vi "CRYUpdate Graph Window.vi"(8 "sOption":string="Update", 9 "Index":i32[](array[numeric]), 10 "Del/Update Names":string[](array[string]), 11 "Type":enum16{"Curves", "Values", "Results", "WFM"}(ring)) -> ()   [LabVIEW 2013]
uses:
  CRYCurveLibrary/Global/CRYCurve Library Global.vi
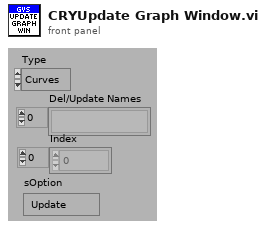
[diagram p1: front panel]
types:
  T1 = cluster{"Curve Index":i32[], "Value Index":i32[], "Result Index":i32[], "WFM Index":i32[], "Curve Names":string[], "Value Names":string[], "Result Names":string[], "WFM Names":string[]}
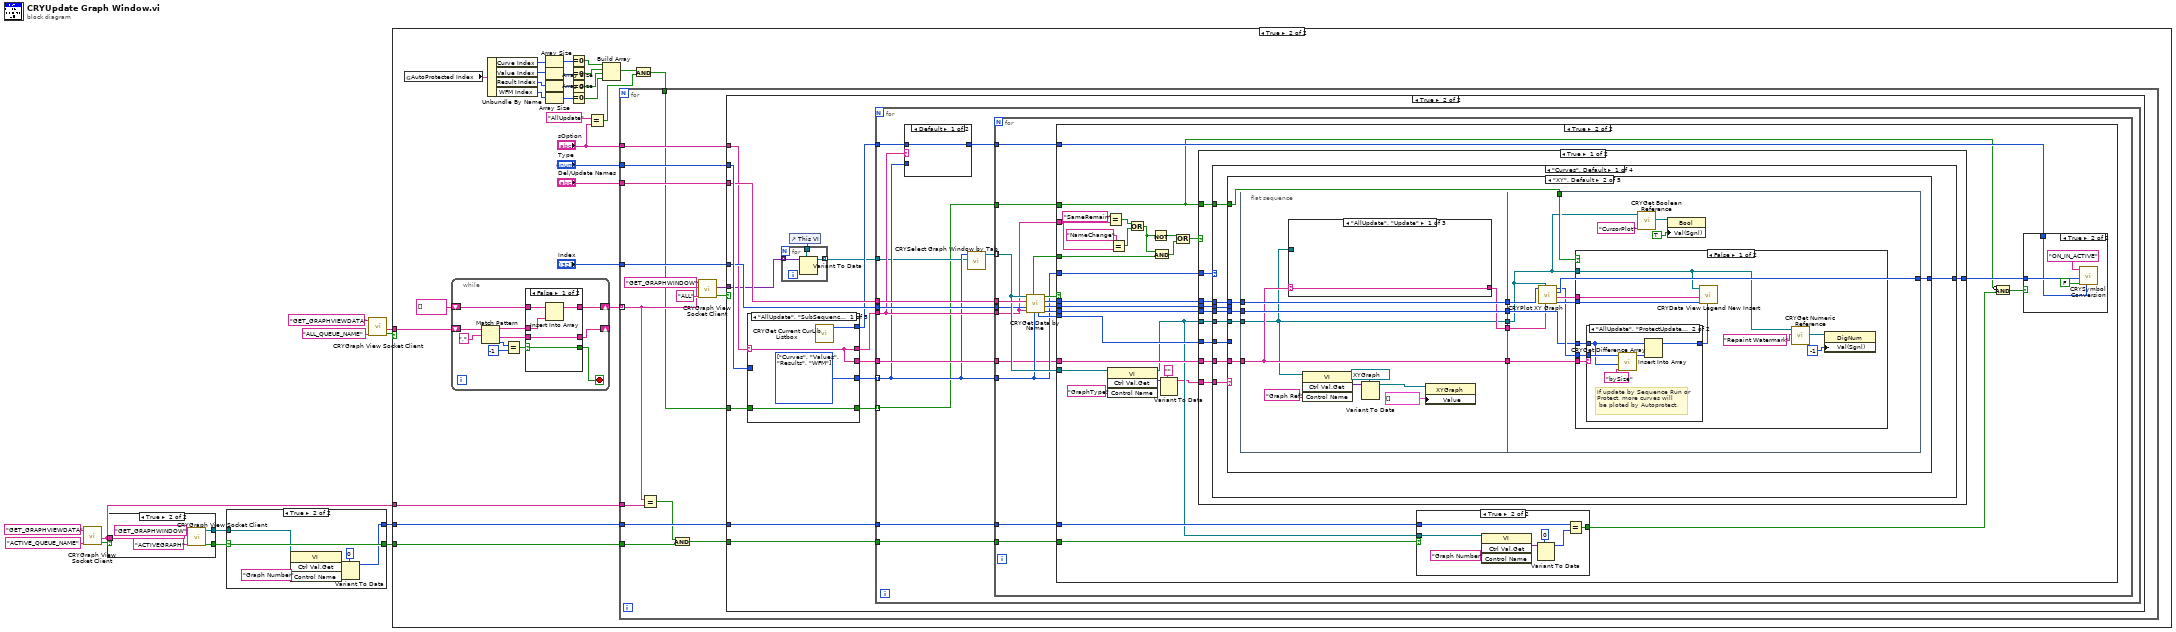
[diagram p0: block diagram]
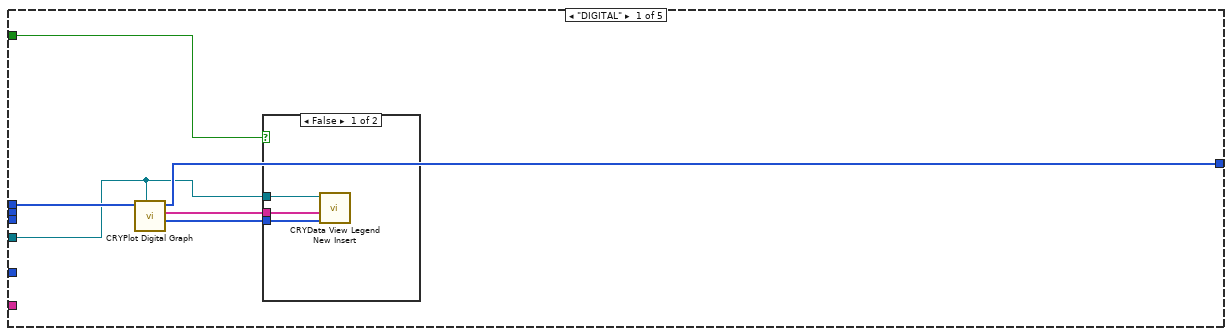
[diagram p10: hidden frame]
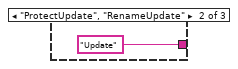
[diagram p12: hidden frame]
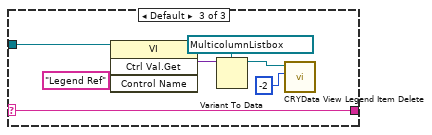
[diagram p13: hidden frame]
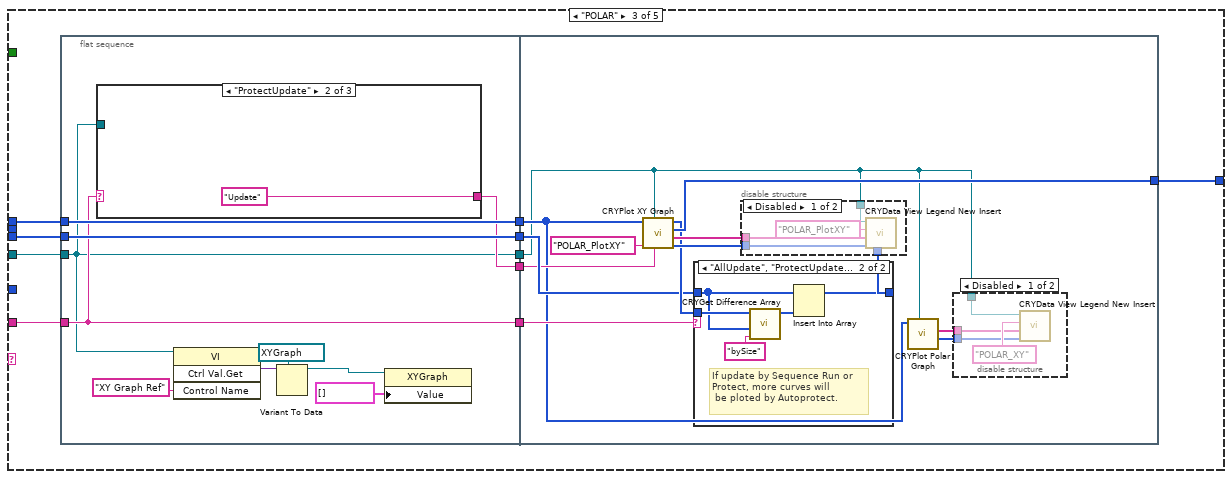
[diagram p16: hidden frame]
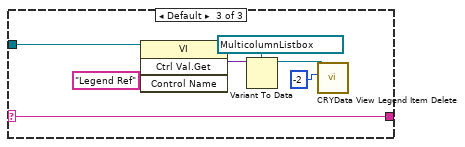
[diagram p18: hidden frame]
diagram:
  n1 = call "CRYGraph View Socket Client.vi"("sOption"="ACTIVE_QUEUE_NAME", "sAction"="GET_GRAPHVIEWDATA") -> ("bResult Out"=w6:bool, "sData Out"=w1:string)  [unwired: 6 in, 2 out]
  n2 = case shown="True" w6 {
    selector: w6 -> [w13 _]
    tunnel: w1 -> [_ w16]
    tunnel: [w13 w15] -> w5
    tunnel: [_ w14] -> w4
    frame False {
    }
    frame True {
      n3 = call "CRYGraph View Socket Client.vi"("sOption"="ACTIVEGRAPH", "sData"=w16, "sAction"="GET_GRAPHWINDOW") -> ("bResult Out"=w15:bool, "pVI Out"=w14:refnum<vi>)  [unwired: 5 in, 2 out]
    }
  }
  n4 = case shown="True" w5 {
    selector: w5 -> [w19 w25]
    tunnel: w4 -> [_ w21]
    tunnel: [_ w20] -> w3
    tunnel: [w19 w25] -> w2
    frame False {
    }
    frame True {
      n5 = invoke class="VI" method="Ctrl Val.Get"(reference=w21, "Control Name"="Graph Number") -> ("Get Control Value Variant"=w23:variant)  [unwired: 2 in, 3 out]
      n6 = Variant To Data(type=0 ("Graph Number"), Variant=w23) -> (data=w20:i32)  [unwired: 1 in, 1 out]
    }
  }
  n7 = call "CRYGraph View Socket Client.vi"("sOption"="ALL_QUEUE_NAME", "sAction"="GET_GRAPHVIEWDATA") -> ("bResult Out"=w10:bool, "sData Out"=w9:string)  [unwired: 6 in, 2 out]
  n8 = case shown="True" w10 {
    tunnel: w9 -> [_ w52]
    tunnel: w3 -> [_ w46]
    tunnel: w2 -> [_ w45]
    tunnel: w1 -> [_ w44]
    frame False {
    }
    frame True {
      n9 = global read "CRYCurve Library Global.vi" "AutoProtected Index"() -> (w34:T1)
      n10 = while {
        shift-right: [w56] -> w50
        shift-left: string[] [] ("Array") -> [w57]
        shift-right: [w53] -> _
        shift-left: w52 -> [w63]
        stop <- w58 stop-if-true
        n11 = Match Pattern(string=w63, regular expression="," ("sOption")) -> (before substring=w55:string, after substring=w54:string, offset past match=w61:i32)  [unwired: 1 in, 1 out]
        n12 = Equal?(x=w61, y=-1) -> (x = y?=w59:bool)
        n13 = case shown="False" w59 {
          selector: w59 -> [w68 w71]
          tunnel: [w68 w71] -> w58
          tunnel: [w65 w70] -> w56
          tunnel: w57 -> [w67 w70]
          tunnel: w55 -> [w66 _]
          tunnel: [w64 w69] -> w53
          tunnel: w54 -> [w64 w69]
          frame False {
            n14 = Insert Into Array(array=w67, new element=w66) -> (w65:string[])  [unwired: 1 in]
          }
          frame True {
          }
        }
      }
      n15 = Unbundle By Name(w34) -> ("Curve Index"=w33:i32[], "Value Index"=w35:i32[], "Result Index"=w36:i32[], "WFM Index"=w37:i32[])
      n16 = Array Size(array=w33) -> (size(s)=w38:i32)
      n17 = Array Size(array=w35) -> (size(s)=w39:i32)
      n18 = Array Size(array=w36) -> (size(s)=w40:i32)
      n19 = Array Size(array=w37) -> (size(s)=w41:i32)
      n20 = Equal To 0?(x=w38) -> (x = 0?=w32:bool)
      n21 = Equal To 0?(x=w39) -> (x = 0?=w31:bool)
      n22 = Equal To 0?(x=w40) -> (x = 0?=w30:bool)
      n23 = Equal To 0?(x=w41) -> (x = 0?=w29:bool)
      n24 = Equal?(x="AllUpdate", y="sOption") -> (x = y?=w27:bool)
      n25 = Build Array(w32, w31, w30, w29) -> (w28:bool[])
      n26 = And(x=w28, y=w27) -> (x .and. y?=w26:bool[])
      n27 = for {
        tunnel: w50 -> [w77] mode=indexing
        tunnel: "Type" -> [w82]
        tunnel: "Del/Update Names" -> [w81]
        tunnel: "Index" -> [w80]
        tunnel: "sOption" -> [w79]
        tunnel: w46 -> [w78]
        tunnel: w45 -> [w74]
        tunnel: w44 -> [w76]
        tunnel: w26 -> [w72]
        n28 = Equal?(x=w77, y=w76) -> (x = y?=w75:bool)
        n29 = And(x=w75, y=w74) -> (x .and. y?=w73:bool)
        n30 = call "CRYGraph View Socket Client.vi"("sOption"="ALL", "sData"=w77, "sAction"="GET_GRAPHWINDOW") -> ("bResult Out"=w83:bool, "Variant Out"=w84:variant[])  [unwired: 5 in, 2 out]
        n31 = case shown="True" w83 {
          tunnel: w84 -> [_ w90]
          tunnel: w82 -> [_ w101]
          tunnel: w81 -> [_ w100]
          tunnel: w80 -> [_ w99]
          tunnel: w79 -> [_ w96]
          tunnel: w78 -> [_ w98]
          tunnel: w73 -> [_ w97]
          tunnel: w72 -> [_ w88]
          frame False {
          }
          frame True {
            n32 = case shown="\"AllUpdate\", \"SubSequenceRemoveUpdate\"" w96 {
              selector: w96 -> [w623 w629 _ w636 w641]
              tunnel: w101 -> [_ w628 w632 w637 w642]
              tunnel: [w623 w629 w631 w636 "GetByName"] -> w95
              tunnel: [w625 w627 w633 w638 w643] -> w94
              tunnel: [w624 w628 w632 w637 w642] -> w93
              tunnel: [w623 w629 w631 "Update" w641] -> w92
              tunnel: w88 -> [w622 _ _ _ _]
              tunnel: [w622 bool[] [FALSE] bool[] [FALSE] bool[] [FALSE] bool[] [FALSE]] -> w87
              frame "AllUpdate", "SubSequenceRemoveUpdate" {
                w625 = enum16{"Curves", "Values", "Results", "WFM"}[] [enum."Curves", enum."Values", enum."Results", enum."WFM"] items=["Curves", "Values", "Results", "WFM"]
                n33 = call "CRYGet Current CurLib Listbox.vi"() -> ("Type"=w624:enum16{"Curves", "Values", "Results", "WFM"})  [unwired: 9 in, 2 out]
              }
              frame "Apply", "ProtectUpdate", "RenameUpdate" {
                n34 = Build Array(w628) -> (w627:enum16{"Curves", "Values", "Results", "WFM"}[])
              }
              frame Default {
                w631 = "GetByName"
                n35 = Build Array(w632) -> (w633:enum16{"Curves", "Values", "Results", "WFM"}[])
              }
              frame "NameChange", "SameRemain" {
                n36 = Build Array(w637) -> (w638:enum16{"Curves", "Values", "Results", "WFM"}[])
              }
              frame "Update" {
                n37 = Build Array(w642) -> (w643:enum16{"Curves", "Values", "Results", "WFM"}[])
              }
            }
            n38 = control-ref of="This VI"() -> (w91:refnum<vi>)
            n39 = for {
              tunnel: w90 -> [w104] mode=indexing
              tunnel: w91 -> [w103]
              tunnel: [w102] -> w89 mode=indexing
              n40 = Variant To Data(type=w103, Variant=w104) -> (data=w102:refnum<vi>)  [unwired: 1 in, 1 out]
            }
            n41 = for {
              tunnel: w100 -> [w116]
              tunnel: w99 -> [w115]
              tunnel: w98 -> [w114]
              tunnel: w97 -> [w113]
              tunnel: w95 -> [w110]
              tunnel: w94 -> [w109] mode=indexing
              tunnel: w93 -> [w108]
              tunnel: w92 -> [w111]
              tunnel: w89 -> [w106]
              tunnel: w87 -> [w105] mode=indexing
              n42 = case shown="Default" w110 {
                tunnel: w109 -> [_ w118]
                tunnel: w108 -> [w117 _]
                tunnel: [w117 w118] -> w107
                frame Default {
                }
                frame "AllUpdate", "SubSequenceRemoveUpdate" {
                }
              }
              n43 = call "CRYSelect Graph Window by Tab.vi"("pGraph VIs In"=w106, "Type"=w109) -> ("pGraph VIs Out"=w112:refnum<vi>[])  [unwired: 9 in]
              n44 = for {
                tunnel: w116 -> [w134]
                tunnel: w112 -> [w130] mode=indexing
                tunnel: w109 -> [w123]
                tunnel: w115 -> [w127]
                tunnel: w110 -> [w120]
                tunnel: w114 -> [w126]
                tunnel: w113 -> [w125]
                tunnel: w107 -> [w124]
                tunnel: w111 -> [w122]
                tunnel: w105 -> [w119]
                n45 = call "CRYGet Data by Name.vi"("Type"=w123, "sOption"=w120, "AutoProtected Index"=w127, "Data Names"=w134, "pVIGraph In"=w130) -> ("Item Symbols"=w131:i32[], "Value Rows"=w132:i32[], "Curve Rows"=w133:i32[], "Replot?"=w129:bool, "Result Rows"=w128:i32[], "bSameRemainReplot"=w121:bool)  [unwired: 1 out]
                n46 = case shown="True" w129 {
                  tunnel: w133 -> [_ w163]
                  tunnel: w132 -> [_ w162]
                  tunnel: w131 -> [_ w161]
                  tunnel: w130 -> [_ w140]
                  tunnel: w123 -> [_ w155]
                  tunnel: w128 -> [_ w160]
                  tunnel: w126 -> [_ w157]
                  tunnel: w125 -> [_ w158]
                  tunnel: w124 -> [_ w156]
                  tunnel: w122 -> [_ w154]
                  tunnel: w121 -> [_ w152]
                  tunnel: w120 -> [_ w149]
                  tunnel: w119 -> [_ w135]
                  frame False {
                  }
                  frame True {
                    n47 = Equal?(x="SameRemain", y=w149) -> (x = y?=w148:bool)
                    n48 = invoke class="VI" method="Ctrl Val.Get"(reference=w140, "Control Name"="GraphType") -> (reference out=w139:refnum<vi>, "Get Control Value Variant"=w143:variant)  [unwired: 2 in, 2 out]
                    n49 = Equal?(x="NameChange", y=w149) -> (x = y?=w147:bool)
                    n50 = Or(x=w148, y=w147) -> (x .or. y?=w146:bool)
                    n51 = Not(x=w146) -> (.not. x?=w144:bool)
                    n52 = And(x=w146, y=w152) -> (x .and. y?=w145:bool)
                    n53 = Variant To Data(type="", Variant=w143) -> (data=w138:string)  [unwired: 1 in, 1 out]
                    n54 = Or(x=w144, y=w145) -> (x .or. y?=w151:bool)
                    n55 = case shown="True" w151 {
                      tunnel: w163 -> [w181 w606]
                      tunnel: w162 -> [w180 w605]
                      tunnel: w161 -> [w179 _]
                      tunnel: w160 -> [w178 w604]
                      tunnel: w138 -> [w177 w608]
                      tunnel: [w176 w603] -> w159
                      tunnel: w139 -> [w175 _]
                      tunnel: w155 -> [w174 w607]
                      tunnel: w154 -> [w173 _]
                      tunnel: w135 -> [w172 _]
                      frame True {
                        n56 = case shown="\"Curves\", Default" w174 {
                          tunnel: w177 -> [w190 _ w442 w488]
                          tunnel: w181 -> [w189 w412 w443 w491]
                          tunnel: w180 -> [w188 w413 w441 _]
                          tunnel: w179 -> [w187 _ _ w486]
                          tunnel: w178 -> [w186 w411 w440 _]
                          tunnel: [w185 w409 w439 w490] -> w176
                          tunnel: w175 -> [w184 w404 w438 w489]
                          tunnel: w173 -> [w183 _ _ w487]
                          tunnel: w172 -> [w182 w403 w437 w485]
                          frame "Curves", Default {
                            n57 = case shown="\"XY\", Default" w190 {
                              tunnel: w189 -> [w196 w209 w267 w325 w379]
                              tunnel: w188 -> [_ _ _ _ w378]
                              tunnel: w187 -> [_ w210 w268 w317 _]
                              tunnel: w186 -> [_ _ _ _ w377]
                              tunnel: [w193 w206 w264 w323 w376] -> w185
                              tunnel: w184 -> [w192 w205 w263 w322 w370]
                              tunnel: w183 -> [_ w203 w262 w319 _]
                              tunnel: w182 -> [w191 w200 _ w316 w369]
                              frame "DIGITAL" {
                                n58 = call "CRYPlot Digital Graph.vi"("pGraph VI In"=w192, "Selected Row In"=w196) -> ("Color Info"=w194:u32[], "Curve Name"=w195:string[], "Selected Row Out"=w193:i32[])  [unwired: 7 out]
                                n59 = case shown="False" w191 {
                                tunnel: w195 -> [w199 _]
                                tunnel: w194 -> [w198 _]
                                tunnel: w192 -> [w197 _]
                                frame False {
                                n60 = call "CRYData View Legend New Insert.vi"("Color Array"=w198, "ItemName Array"=w199, "pGraph VI In"=w197) -> ()  [unwired: 2 in, 7 out]
                                }
                                frame True {
                                }
                                }
                              }
                              frame "XY", Default {
                                n61 = flat-sequence {
                                tunnel: w209 -> [w219]
                                tunnel: w210 -> [w220]
                                tunnel: [w220] -> w208
                                tunnel: [w219] -> w207
                                tunnel: w205 -> [w212]
                                tunnel: [w212] -> w204
                                tunnel: w203 -> [w216]
                                tunnel: [w216] -> w202
                                tunnel: [w217] -> w201
                                tunnel: [w242] -> w206
                                tunnel: w200 -> [w234]
                                tunnel: w201 -> [w236]
                                tunnel: w202 -> [w235]
                                tunnel: w204 -> [w230]
                                tunnel: w207 -> [w239]
                                tunnel: w208 -> [w237]
                                frame #0 {
                                n62 = case shown="\"AllUpdate\", \"Update\"" w216 {
                                selector: w216 -> [w221 _ w228]
                                tunnel: [w221 "Update" w228] -> w217
                                tunnel: w212 -> [_ _ w223]
                                frame "AllUpdate", "Update" {
                                }
                                frame "ProtectUpdate", "RenameUpdate" {
                                }
                                frame Default {
                                n63 = invoke class="VI" method="Ctrl Val.Get"(reference=w223, "Control Name"="Legend Ref") -> ("Get Control Value Variant"=w226:variant)  [unwired: 2 in, 3 out]
                                n64 = Variant To Data(type=refnum<vi> refnum ("GMListbox"), Variant=w226) -> (data=w224:refnum<vi>)  [unwired: 1 in, 1 out]
                                n65 = call "CRYData View Legend Item Delete.vi"("RowNumber"=-2, "Legend MultiListbox In"=w224) -> ()  [unwired: 10 out]
                                }
                                }
                                n66 = invoke class="VI" method="Ctrl Val.Get"(reference=w212, "Control Name"="Graph Ref") -> ("Get Control Value Variant"=w215:variant)  [unwired: 2 in, 3 out]
                                n67 = Variant To Data(type=refnum<vi> refnum ("XY Graph"), Variant=w215) -> (data=w211:refnum<vi>)  [unwired: 1 in, 1 out]
                                n68 = property class="XYGraph"(reference=w211, "Value"=cluster{"XY Graph":cluster{dbl, dbl}[]}[] [] ("XY Graph")) -> ()  [unwired: 1 in, 2 out]
                                }
                                frame #1 {
                                n69 = call "CRYPlot XY Graph.vi"("sOption"=w236, "pGraph VI In"=w230, "Selected Rows In"=w239) -> ("Color Info"=w240:u32[], "Curve Name"=w241:string[], "All Rows Out"=w242:i32[], "ItemSyms"=w238:i32[])  [unwired: 3 in, 2 out]
                                n70 = case shown="False" w234 {
                                tunnel: w241 -> [w249 _]
                                tunnel: w240 -> [w248 _]
                                tunnel: w238 -> [w247 _]
                                tunnel: w237 -> [w246 _]
                                tunnel: w235 -> [w245 _]
                                tunnel: w230 -> [w243 _]
                                frame False {
                                n71 = case shown="\"AllUpdate\", \"ProtectUpdate\"" w245 {
                                tunnel: w247 -> [w253 w256]
                                tunnel: w246 -> [_ w255]
                                tunnel: [w253 w254] -> w244
                                frame Default {
                                }
                                frame "AllUpdate", "ProtectUpdate" {
                                # "If update by Sequence Run or\nProtect, more curves will\n be ploted by Autoprotect."
                                n72 = call "CRYGet Difference Array.vi"("sOption"="bySize", "Array 2"=w255, "Array 1"=w256) -> ("Diff Out"=w258:i32[])  [unwired: 7 in, 1 out]
                                n73 = Insert Into Array(array=w255, new element=w258) -> (w254:i32[])  [unwired: 1 in]
                                }
                                }
                                n74 = call "CRYData View Legend New Insert.vi"("Item Symbols"=w244, "Color Array"=w248, "ItemName Array"=w249, "pGraph VI In"=w243) -> ()  [unwired: 1 in, 7 out]
                                n75 = call "CRYGet Numeric Reference.vi"("Label Name"="Repaint Watermark", "VI Refnum"=w243) -> ("Numeric Ref Out"=w251:refnum<vi>)  [unwired: 7 in, 2 out]
                                n76 = property class="DigNum"(reference=w251, "Val(Sgnl)"=-1 ("y")) -> ()  [unwired: 1 in, 2 out]
                                }
                                frame True {
                                }
                                }
                                n77 = call "CRYGet Boolean Reference.vi"("Label Name"="CursorPlot", "VI Refnum"=w230) -> ("Boolean Ref"=w233:refnum<vi>)  [unwired: 7 in, 2 out]
                                n78 = property class="Bool"(reference=w233, "Val(Sgnl)"=TRUE) -> ()  [unwired: 1 in, 2 out]
                                }
                                }
                              }
                              frame "POLAR" {
                                n79 = flat-sequence {
                                tunnel: w267 -> [w277]
                                tunnel: w268 -> [w278]
                                tunnel: [w278] -> w266
                                tunnel: [w277] -> w265
                                tunnel: w263 -> [w269]
                                tunnel: w262 -> [w274]
                                tunnel: [w274] -> w261
                                tunnel: [w275] -> w260
                                tunnel: [w269] -> w259
                                tunnel: [w300] -> w264
                                tunnel: w260 -> [w294]
                                tunnel: w261 -> [w293]
                                tunnel: w265 -> [w290]
                                tunnel: w266 -> [w296]
                                tunnel: w259 -> [w289]
                                frame #0 {
                                n80 = case shown="\"ProtectUpdate\"" w274 {
                                selector: w274 -> [w279 _ w286]
                                tunnel: [w279 "Update" w286] -> w275
                                tunnel: w269 -> [_ _ w281]
                                frame "AllUpdate", "Update" {
                                }
                                frame "ProtectUpdate" {
                                }
                                frame Default {
                                n81 = invoke class="VI" method="Ctrl Val.Get"(reference=w281, "Control Name"="Legend Ref") -> ("Get Control Value Variant"=w284:variant)  [unwired: 2 in, 3 out]
                                n82 = Variant To Data(type=refnum<vi> refnum ("GMListbox"), Variant=w284) -> (data=w282:refnum<vi>)  [unwired: 1 in, 1 out]
                                n83 = call "CRYData View Legend Item Delete.vi"("RowNumber"=-2, "Legend MultiListbox In"=w282) -> ()  [unwired: 10 out]
                                }
                                }
                                n84 = invoke class="VI" method="Ctrl Val.Get"(reference=w269, "Control Name"="XY Graph Ref") -> ("Get Control Value Variant"=w273:variant)  [unwired: 2 in, 3 out]
                                n85 = Variant To Data(type=refnum<vi> refnum ("XY Graph"), Variant=w273) -> (data=w270:refnum<vi>)  [unwired: 1 in, 1 out]
                                n86 = property class="XYGraph"(reference=w270, "Value"=cluster{"XY Graph":cluster{dbl, dbl}[]}[] [] ("XY Graph")) -> ()  [unwired: 1 in, 2 out]
                                }
                                frame #1 {
                                n87 = call "CRYPlot XY Graph.vi"("sOption"=w294, "pGraph VI In"=w289, "sType"="POLAR_PlotXY" ("sOption"), "Selected Rows In"=w290) -> ("Color Info"=w298:u32[], "Curve Name"=w299:string[], "All Rows Out"=w300:i32[], "ItemSyms"=w297:i32[])  [unwired: 2 in, 2 out]
                                n88 = case shown="\"AllUpdate\", \"ProtectUpdate\"" w293 {
                                tunnel: w297 -> [w310 w313]
                                tunnel: w296 -> [_ w312]
                                tunnel: [w310 w311] -> w295
                                frame Default {
                                }
                                frame "AllUpdate", "ProtectUpdate" {
                                # "If update by Sequence Run or\nProtect, more curves will\n be ploted by Autoprotect."
                                n89 = call "CRYGet Difference Array.vi"("sOption"="bySize", "Array 2"=w312, "Array 1"=w313) -> ("Diff Out"=w315:i32[])  [unwired: 7 in, 1 out]
                                n90 = Insert Into Array(array=w312, new element=w315) -> (w311:i32[])  [unwired: 1 in]
                                }
                                }
                                n91 = disable-structure shown="Disabled" {
                                disable-tunnel: w299 -> [w305 _]
                                disable-tunnel: w298 -> [w304 _]
                                disable-tunnel: w295 -> [w303 _]
                                disable-tunnel: w289 -> [w301 _]
                                frame Disabled {
                                n92 = call "CRYData View Legend New Insert.vi"("Item Symbols"=w303, "Color Array"=w304, "ItemName Array"=w305, "sOption"="POLAR_PlotXY", "pGraph VI In"=w301) -> ()  [unwired: 7 out]
                                }
                                frame Enabled {
                                }
                                }
                                n93 = call "CRYPlot Polar Graph.vi"("pGraph VI In"=w289, "Selected Rows In"=w290) -> ("Freq Color"=w292:u32[], "Freq Name"=w291:string[])  [unwired: 4 in, 4 out]
                                n94 = disable-structure shown="Disabled" {
                                disable-tunnel: w292 -> [w308 _]
                                disable-tunnel: w291 -> [w307 _]
                                disable-tunnel: w289 -> [w306 _]
                                frame Disabled {
                                n95 = call "CRYData View Legend New Insert.vi"("Color Array"=w308, "ItemName Array"=w307, "sOption"="POLAR_XY", "pGraph VI In"=w306) -> ()  [unwired: 1 in, 7 out]
                                }
                                frame Enabled {
                                }
                                }
                                }
                                }
                              }
                              frame "OCTAVE" {
                                n96 = flat-sequence {
                                tunnel: w325 -> [w334]
                                tunnel: [w334] -> w324
                                tunnel: w322 -> [w326]
                                tunnel: [w326] -> w321
                                tunnel: [w332] -> w320
                                tunnel: w319 -> [w332]
                                tunnel: [w331] -> w318
                                tunnel: w317 -> [w331]
                                tunnel: [w352] -> w323
                                tunnel: w316 -> [w345]
                                tunnel: w318 -> [w348]
                                tunnel: w320 -> [w347]
                                tunnel: w321 -> [w341]
                                tunnel: w324 -> [w349]
                                frame #0 {
                                n97 = case shown="Default" w332 {
                                tunnel: w326 -> [_ w335]
                                frame "AllUpdate", "ProtectUpdate", "Update" {
                                }
                                frame Default {
                                n98 = invoke class="VI" method="Ctrl Val.Get"(reference=w335, "Control Name"="Legend Ref") -> ("Get Control Value Variant"=w339:variant)  [unwired: 2 in, 3 out]
                                n99 = Variant To Data(type=refnum<vi> refnum ("GMListbox"), Variant=w339) -> (data=w336:refnum<vi>)  [unwired: 1 in, 1 out]
                                n100 = call "CRYData View Legend Item Delete.vi"("RowNumber"=-2, "Legend MultiListbox In"=w336) -> ()  [unwired: 10 out]
                                }
                                }
                                n101 = invoke class="VI" method="Ctrl Val.Get"(reference=w326, "Control Name"="Graph Ref") -> ("Get Control Value Variant"=w330:variant)  [unwired: 2 in, 3 out]
                                n102 = Variant To Data(type=refnum<vi> refnum ("XY Graph"), Variant=w330) -> (data=w327:refnum<vi>)  [unwired: 1 in, 1 out]
                                n103 = property class="XYGraph"(reference=w327, "Value"=cluster{"XY Graph":cluster{dbl, dbl}[]}[] [] ("XY Graph")) -> ()  [unwired: 1 in, 2 out]
                                }
                                frame #1 {
                                n104 = call "CRYPlot Octave Graph.vi"("sOption"=w347, "pGraph VI In"=w341, "Selected Rows In"=w349) -> ("Color Info"=w350:u32[], "Curve Name"=w351:string[], "All Rows Out"=w352:i32[], "ItemSyms"=w346:i32[])  [unwired: 5 in]
                                n105 = case shown="False" w345 {
                                tunnel: w351 -> [w359 _]
                                tunnel: w350 -> [w358 _]
                                tunnel: w348 -> [w357 _]
                                tunnel: w347 -> [w356 _]
                                tunnel: w341 -> [w353 _]
                                tunnel: w346 -> [w355 _]
                                frame False {
                                n106 = case shown="\"AllUpdate\", \"ProtectUpdate\"" w356 {
                                tunnel: [w363 w366] -> w354
                                tunnel: w357 -> [_ w365]
                                tunnel: w355 -> [w363 w364]
                                frame "False", Default {
                                }
                                frame "AllUpdate", "ProtectUpdate" {
                                # "If update by Sequence Run or\nProtect, more curves will\n be ploted by Autoprotect."
                                n107 = call "CRYGet Difference Array.vi"("sOption"="bySize", "Array 2"=w365, "Array 1"=w364) -> ("Diff Out"=w368:i32[])  [unwired: 7 in, 1 out]
                                n108 = Insert Into Array(array=w365, new element=w368) -> (w366:i32[])  [unwired: 1 in]
                                }
                                }
                                n109 = call "CRYData View Legend New Insert.vi"("Item Symbols"=w354, "Color Array"=w358, "ItemName Array"=w359, "pGraph VI In"=w353) -> ()  [unwired: 1 in, 7 out]
                                n110 = call "CRYGet Numeric Reference.vi"("Label Name"="Repaint Watermark", "VI Refnum"=w353) -> ("Numeric Ref Out"=w361:refnum<vi>)  [unwired: 7 in, 2 out]
                                n111 = property class="DigNum"(reference=w361, "Val(Sgnl)"=-1 ("y")) -> ()  [unwired: 1 in, 2 out]
                                }
                                frame True {
                                }
                                }
                                n112 = call "CRYGet Boolean Reference.vi"("Label Name"="CursorPlot", "VI Refnum"=w341) -> ("Boolean Ref"=w342:refnum<vi>)  [unwired: 7 in, 2 out]
                                n113 = property class="Bool"(reference=w342, "Val(Sgnl)"=TRUE) -> ()  [unwired: 1 in, 2 out]
                                }
                                }
                              }
                              frame "TABLE" {
                                n114 = call "CRYPlot Table.vi"("Result Rows In"=w377, "pGraph VI In"=w370, "Value Rows In"=w378, "Curve Rows In"=w379) -> ("Value Name"=w372:string[], "Value Rows Out"=w375:i32[], "Curve Name"=w373:string[], "Curve Rows Out"=w376:i32[], "Result Rows Out"=w374:i32[], "Result Name"=w371:string[])  [unwired: 2 in]
                                n115 = case shown="False" w369 {
                                tunnel: w375 -> [w385 _]
                                tunnel: w374 -> [w384 _]
                                tunnel: w373 -> [w383 _]
                                tunnel: w372 -> [w382 _]
                                tunnel: w371 -> [w381 _]
                                tunnel: w370 -> [w380 _]
                                frame False {
                                n116 = flat-sequence {
                                tunnel: w384 -> [w393]
                                tunnel: w385 -> [w394]
                                tunnel: [w394] -> w387
                                tunnel: [w393] -> w386
                                tunnel: w383 -> [w391]
                                tunnel: w382 -> [w390]
                                tunnel: w381 -> [w389]
                                tunnel: w380 -> [w388]
                                tunnel: w387 -> [w400]
                                tunnel: w386 -> [w395]
                                frame #0 {
                                n117 = Insert Into Array(array=w391, new element #1=w390, new element #2=w389) -> (w392:string[])  [unwired: 1 in]
                                n118 = call "CRYData View Legend New Insert.vi"("ItemName Array"=w392, "pGraph VI In"=w388) -> ()  [unwired: 3 in, 7 out]
                                }
                                frame #1 {
                                n119 = call "CRYSymbol Conversion.vi"("CurLib Tab Type"=enum16{"Curves", "Values", "Results", "WFM"}."Values", "bData"=FALSE, "nDatas"=w400, "sActin"="ON_IN_ACTIVE") -> ()  [unwired: 8 in]
                                n120 = call "CRYSymbol Conversion.vi"("CurLib Tab Type"=enum16{"Curves", "Values", "Results", "WFM"}."Results", "bData"=FALSE, "nDatas"=w395, "sActin"="ON_IN_ACTIVE") -> ()  [unwired: 8 in]
                                }
                                }
                                }
                                frame True {
                                }
                                }
                              }
                            }
                          }
                          frame "Values" {
                            n121 = call "CRYPlot Table.vi"("Result Rows In"=w411, "pGraph VI In"=w404, "Value Rows In"=w413, "Curve Rows In"=w412) -> ("Value Name"=w406:string[], "Value Rows Out"=w409:i32[], "Curve Name"=w407:string[], "Curve Rows Out"=w408:i32[], "Result Rows Out"=w410:i32[], "Result Name"=w405:string[])  [unwired: 2 in]
                            n122 = case shown="False" w403 {
                              tunnel: w410 -> [w419 _]
                              tunnel: w408 -> [w418 _]
                              tunnel: w407 -> [w417 _]
                              tunnel: w406 -> [w416 _]
                              tunnel: w405 -> [w415 _]
                              tunnel: w404 -> [w414 _]
                              frame False {
                                n123 = flat-sequence {
                                tunnel: w418 -> [w427]
                                tunnel: w419 -> [w428]
                                tunnel: [w428] -> w421
                                tunnel: [w427] -> w420
                                tunnel: w417 -> [w425]
                                tunnel: w416 -> [w424]
                                tunnel: w415 -> [w423]
                                tunnel: w414 -> [w422]
                                tunnel: w421 -> [w430]
                                tunnel: w420 -> [w429]
                                frame #0 {
                                n124 = Insert Into Array(array=w425, new element #1=w424, new element #2=w423) -> (w426:string[])  [unwired: 1 in]
                                n125 = call "CRYData View Legend New Insert.vi"("ItemName Array"=w426, "pGraph VI In"=w422) -> ()  [unwired: 3 in, 7 out]
                                }
                                frame #1 {
                                n126 = call "CRYSymbol Conversion.vi"("CurLib Tab Type"=enum16{"Curves", "Values", "Results", "WFM"}."Curves", "bData"=FALSE, "nDatas"=w429, "sActin"="ON_IN_ACTIVE") -> ()  [unwired: 8 in]
                                n127 = call "CRYSymbol Conversion.vi"("CurLib Tab Type"=enum16{"Curves", "Values", "Results", "WFM"}."Results", "bData"=FALSE, "nDatas"=w430, "sActin"="ON_IN_ACTIVE") -> ()  [unwired: 8 in]
                                }
                                }
                              }
                              frame True {
                              }
                            }
                          }
                          frame "Results" {
                            n128 = case shown="\"TABLE\"" w442 {
                              tunnel: w443 -> [w454 w482]
                              tunnel: w441 -> [w453 _]
                              tunnel: w440 -> [w452 _]
                              tunnel: [w451 w481] -> w439
                              tunnel: w438 -> [w445 w479]
                              tunnel: w437 -> [w444 w478]
                              frame "TABLE" {
                                n129 = call "CRYPlot Table.vi"("Result Rows In"=w452, "pGraph VI In"=w445, "Value Rows In"=w453, "Curve Rows In"=w454) -> ("Value Name"=w447:string[], "Value Rows Out"=w449:i32[], "Curve Name"=w448:string[], "Curve Rows Out"=w450:i32[], "Result Rows Out"=w451:i32[], "Result Name"=w446:string[])  [unwired: 2 in]
                                n130 = case shown="False" w444 {
                                tunnel: w450 -> [w460 _]
                                tunnel: w449 -> [w459 _]
                                tunnel: w448 -> [w458 _]
                                tunnel: w447 -> [w457 _]
                                tunnel: w446 -> [w456 _]
                                tunnel: w445 -> [w455 _]
                                frame False {
                                n131 = flat-sequence {
                                tunnel: w459 -> [w468]
                                tunnel: w460 -> [w469]
                                tunnel: [w469] -> w462
                                tunnel: [w468] -> w461
                                tunnel: w458 -> [w466]
                                tunnel: w457 -> [w465]
                                tunnel: w456 -> [w464]
                                tunnel: w455 -> [w463]
                                tunnel: w462 -> [w471]
                                tunnel: w461 -> [w470]
                                frame #0 {
                                n132 = Insert Into Array(array=w466, new element #1=w465, new element #2=w464) -> (w467:string[])  [unwired: 1 in]
                                n133 = call "CRYData View Legend New Insert.vi"("ItemName Array"=w467, "pGraph VI In"=w463) -> ()  [unwired: 3 in, 7 out]
                                }
                                frame #1 {
                                n134 = call "CRYSymbol Conversion.vi"("CurLib Tab Type"=enum16{"Curves", "Values", "Results", "WFM"}."Curves", "bData"=FALSE, "nDatas"=w471, "sActin"="ON_IN_ACTIVE") -> ()  [unwired: 8 in]
                                n135 = call "CRYSymbol Conversion.vi"("CurLib Tab Type"=enum16{"Curves", "Values", "Results", "WFM"}."Values", "bData"=FALSE, "nDatas"=w470, "sActin"="ON_IN_ACTIVE") -> ()  [unwired: 8 in]
                                }
                                }
                                }
                                frame True {
                                }
                                }
                              }
                              frame "RESULT", Default {
                                n136 = call "CRYPlot Result.vi"("pGraph VI In"=w479, "Old Rows In"=w482) -> ("Curve Name"=w480:string[], "Selected Rows Out"=w481:i32[])  [unwired: 4 in, 4 out]
                                n137 = case shown="False" w478 {
                                tunnel: w480 -> [w484 _]
                                tunnel: w479 -> [w483 _]
                                frame False {
                                n138 = call "CRYData View Legend New Insert.vi"("ItemName Array"=w484, "pGraph VI In"=w483) -> ()  [unwired: 3 in, 7 out]
                                }
                                frame True {
                                }
                                }
                              }
                            }
                          }
                          frame "WFM" {
                            n139 = case shown="\"WAVE\", Default" w488 {
                              tunnel: w491 -> [w501 w567]
                              tunnel: [w500 w566] -> w490
                              tunnel: w489 -> [w499 w565]
                              tunnel: w487 -> [w497 w564]
                              tunnel: w486 -> [w495 _]
                              tunnel: w485 -> [w492 w563]
                              frame "WAVE", Default {
                                n140 = flat-sequence {
                                tunnel: w501 -> [w518]
                                tunnel: [w518] -> w503
                                tunnel: [w507] -> w502
                                tunnel: w499 -> [w507]
                                tunnel: [w516] -> w498
                                tunnel: w497 -> [w516]
                                tunnel: [w515] -> w496
                                tunnel: w495 -> [w515]
                                tunnel: [w510] -> w494
                                tunnel: [w504] -> w493
                                tunnel: [w536] -> w500
                                tunnel: w492 -> [w527]
                                tunnel: w493 -> [w534]
                                tunnel: w494 -> [w535]
                                tunnel: w496 -> [w530]
                                tunnel: w498 -> [w529]
                                tunnel: w502 -> [w523]
                                tunnel: w503 -> [w531]
                                frame #0 {
                                n141 = invoke class="VI" method="Ctrl Val.Get"(reference=w507, "Control Name"="Graph Ref") -> ("Get Control Value Variant"=w514:variant)  [unwired: 2 in, 3 out]
                                n142 = invoke class="VI" method="Ctrl Val.Get"(reference=w507, "Control Name"="Legend Ref") -> ("Get Control Value Variant"=w509:variant)  [unwired: 2 in, 3 out]
                                n143 = Variant To Data(type=refnum<vi> refnum ("WaveGraph Ref"), Variant=w514) -> (data=w511:refnum<vi>)  [unwired: 1 in, 1 out]
                                n144 = Variant To Data(type=refnum<vi> refnum ("GMListbox"), Variant=w509) -> (data=w505:refnum<vi>)  [unwired: 1 in, 1 out]
                                n145 = property class="WFGraph"(reference=w511, "Value"=cluster{"xo":dbl, "dx":dbl, dbl[]}[] [] ("WaveGraph")) -> (reference out=w504:refnum<vi>)  [unwired: 1 in, 1 out]
                                n146 = case shown="\"AllUpdate\", \"ProtectUpdate\", \"Update\"" w516 {
                                tunnel: [w520 w522] -> w510
                                tunnel: w505 -> [w519 w522]
                                frame Default {
                                n147 = call "CRYData View Legend Item Delete.vi"("RowNumber"=-2, "Legend MultiListbox In"=w519) -> ("Legend MultiListbox Out"=w520:refnum<vi>)  [unwired: 9 out]
                                }
                                frame "AllUpdate", "ProtectUpdate", "Update" {
                                }
                                }
                                }
                                frame #1 {
                                n148 = call "CRYPlot Wave Graph.vi"("sOption"=w529, "pGraph VI In"=w523, "Selected Rows In"=w531) -> ("ItemSyms"=w528:i32[], "Color Info"=w533:u32[], "Curve Name"=w532:string[], "Selected Rows Out"=w536:i32[])  [unwired: 2 in, 3 out]
                                n149 = case shown="False" w527 {
                                tunnel: w535 -> [w552 _]
                                tunnel: w534 -> [w550 _]
                                tunnel: w533 -> [w543 _]
                                tunnel: w532 -> [w542 _]
                                tunnel: w530 -> [w541 _]
                                tunnel: w529 -> [w540 _]
                                tunnel: w528 -> [w539 _]
                                tunnel: w523 -> [w538 _]
                                frame False {
                                n150 = case shown="\"AllUpdate\", \"ProtectUpdate\"" w540 {
                                tunnel: w539 -> [w553 w558]
                                tunnel: w541 -> [_ w557]
                                tunnel: [w553 w555] -> w537
                                frame Default {
                                }
                                frame "AllUpdate", "ProtectUpdate" {
                                # "If update by Sequence Run or\nProtect, more curves will\n be ploted by Autoprotect."
                                n151 = call "CRYGet Difference Array.vi"("sOption"="bySize", "Array 2"=w557, "Array 1"=w558) -> ("Diff Out"=w556:i32[])  [unwired: 7 in, 1 out]
                                n152 = Insert Into Array(array=w557, new element=w556) -> (w555:i32[])  [unwired: 1 in]
                                }
                                }
                                n153 = call "CRYData View Legend New Insert.vi"("Item Symbols"=w537, "Color Array"=w543, "ItemName Array"=w542, "pGraph VI In"=w538) -> ("pGraph VI Out"=w551:refnum<vi>)  [unwired: 1 in, 6 out]
                                n154 = call "CRYGet Legend Name.vi"("MCListbox Refnum"=w552) -> ("Names Out"=w545:string[])  [unwired: 2 in, 8 out]
                                n155 = Array Size(array=w545) -> (size(s)=w546:i32)
                                n156 = case shown="0" w546 {
                                tunnel: w550 -> [w561 _]
                                tunnel: [w559 errorcluster {"status"=FALSE, "code"=0, "source"=""} ("error out")] -> w544
                                frame 0 {
                                n157 = property class="WFGraph"(reference=w561, "Value"=cluster{"xo":dbl, "dx":dbl, dbl[]}[] [{"xo"=0.0, "dx"=0.0, [0.0]}] ("appended array")) -> (error out=w559:errorcluster)  [unwired: 1 in, 1 out]
                                }
                                frame 1, Default {
                                }
                                }
                                n158 = call "CRYGet Numeric Reference.vi"("Label Name"="Repaint Watermark", "VI Refnum"=w551) -> ("Numeric Ref Out"=w548:refnum<vi>)  [unwired: 7 in, 2 out]
                                n159 = property class="DigNum"(reference=w548, error in=w544, "Val(Sgnl)"=-1 ("y")) -> ()  [unwired: 2 out]
                                }
                                frame True {
                                }
                                }
                                n160 = call "CRYGet Boolean Reference.vi"("Label Name"="CursorPlot", "VI Refnum"=w523) -> ("Boolean Ref"=w524:refnum<vi>)  [unwired: 7 in, 2 out]
                                n161 = property class="Bool"(reference=w524, "Val(Sgnl)"=TRUE) -> ()  [unwired: 1 in, 2 out]
                                }
                                }
                              }
                              frame "INTENSITY" {
                                n162 = flat-sequence {
                                tunnel: w567 -> [w578]
                                tunnel: [w578] -> w569
                                tunnel: [w571] -> w568
                                tunnel: w565 -> [w570]
                                tunnel: w564 -> [w576]
                                tunnel: [w594] -> w566
                                tunnel: w568 -> [w585]
                                tunnel: w569 -> [w591]
                                tunnel: w563 -> [w589]
                                frame #0 {
                                n163 = case shown="Default" w576 {
                                tunnel: w570 -> [_ w580]
                                frame "AllUpdate", "Update" {
                                }
                                frame Default {
                                n164 = invoke class="VI" method="Ctrl Val.Get"(reference=w580, "Control Name"="Legend Ref") -> ("Get Control Value Variant"=w582:variant)  [unwired: 2 in, 3 out]
                                n165 = Variant To Data(type=refnum<vi> refnum ("GMListbox"), Variant=w582) -> (data=w579:refnum<vi>)  [unwired: 1 in, 1 out]
                                n166 = call "CRYData View Legend Item Delete.vi"("RowNumber"=-2, "Legend MultiListbox In"=w579) -> ()  [unwired: 10 out]
                                }
                                }
                                n167 = invoke class="VI" method="Ctrl Val.Get"(reference=w570, "Control Name"="Graph Ref") -> (reference out=w571:refnum<vi>, "Get Control Value Variant"=w573:variant)  [unwired: 2 in, 2 out]
                                n168 = Variant To Data(type=refnum<vi> refnum ("Graph Ref"), Variant=w573) -> (data=w572:refnum<vi>)  [unwired: 1 in, 1 out]
                                n169 = property class="IntGraph"(reference=w572, "Value"=dbl[][] [] ("Graph")) -> ()  [unwired: 1 in, 2 out]
                                }
                                frame #1 {
                                n170 = call "CRYPlot Intensity Graph.vi"("pGraph VI In"=w585, "Selected Rows In"=w591) -> ("ItemSyms"=w590:i32[], "Color Info"=w593:u32[], "Wave Names"=w592:string[], "All Rows Out"=w594:i32[])  [unwired: 6 in]
                                n171 = case shown="False" w589 {
                                tunnel: w593 -> [w598 _]
                                tunnel: w592 -> [w597 _]
                                tunnel: w590 -> [w596 _]
                                tunnel: w585 -> [w595 _]
                                frame False {
                                n172 = call "CRYData View Legend New Insert.vi"("Item Symbols"=w596, "Color Array"=w598, "ItemName Array"=w597, "pGraph VI In"=w595) -> ("pGraph VI Out"=w602:refnum<vi>)  [unwired: 1 in, 6 out]
                                n173 = call "CRYGet Numeric Reference.vi"("Label Name"="Repaint Watermark", "VI Refnum"=w602) -> ("Numeric Ref Out"=w600:refnum<vi>)  [unwired: 7 in, 2 out]
                                n174 = property class="DigNum"(reference=w600, "Val(Sgnl)"=-1 ("y")) -> ()  [unwired: 1 in, 2 out]
                                }
                                frame True {
                                }
                                }
                                n175 = call "CRYGet Boolean Reference.vi"("Label Name"="CursorPlot", "VI Refnum"=w585) -> ("Boolean Ref"=w586:refnum<vi>)  [unwired: 7 in, 2 out]
                                n176 = property class="Bool"(reference=w586, "Val(Sgnl)"=TRUE) -> ()  [unwired: 1 in, 2 out]
                                }
                                }
                              }
                            }
                          }
                        }
                      }
                      frame False {
                        n177 = case shown="\"TABLE\"" w608 {
                          tunnel: w607 -> [_ w614]
                          tunnel: [w609 w613] -> w603
                          tunnel: w606 -> [w609 w612]
                          tunnel: w605 -> [_ w611]
                          tunnel: w604 -> [_ w610]
                          frame Default {
                          }
                          frame "TABLE" {
                            n178 = case shown="\"Curves\", Default" w614 {
                              tunnel: [w615 w616 w617] -> w613
                              tunnel: w612 -> [w615 _ _]
                              tunnel: w611 -> [_ w616 _]
                              tunnel: w610 -> [_ _ w617]
                              frame "Curves", Default {
                              }
                              frame "Values" {
                              }
                              frame "Results" {
                              }
                            }
                          }
                        }
                      }
                    }
                    n179 = case shown="True" w158 {
                      selector: w158 -> [w164 _]
                      tunnel: w157 -> [_ w170]
                      tunnel: w139 -> [_ w165]
                      tunnel: [w164 w171] -> w137
                      frame False {
                      }
                      frame True {
                        n180 = invoke class="VI" method="Ctrl Val.Get"(reference=w165, "Control Name"="Graph Number") -> ("Get Control Value Variant"=w168:variant)  [unwired: 2 in, 3 out]
                        n181 = Variant To Data(type=0 ("Graph Number"), Variant=w168) -> (data=w166:i32)  [unwired: 1 in, 1 out]
                        n182 = Equal?(x=w170, y=w166) -> (x = y?=w171:bool)
                      }
                    }
                    n183 = Compound Arithmetic op=AND(invert w135, w137) -> (w136:bool)
                    n184 = case shown="True" w136 {
                      tunnel: w159 -> [_ w621]
                      tunnel: w156 -> [_ w620]
                      frame False {
                      }
                      frame True {
                        n185 = call "CRYSymbol Conversion.vi"("CurLib Tab Type"=w620, "bData"=FALSE, "nDatas"=w621, "sActin"="ON_IN_ACTIVE") -> ()  [unwired: 8 in]
                      }
                    }
                  }
                }
              }
            }
          }
        }
      }
    }
  }
